vi "case.vi"() -> ()   [LabVIEW 2015]
panel:
  out "Numeric 5":dbl
  in  "Numeric 4":dbl
  out "Numeric 3":dbl
  in  "Boolean":bool
  in  "Numeric 2":dbl
  in  "Numeric":dbl
  # "Case §P§O"
  # "Case §P§O 2"
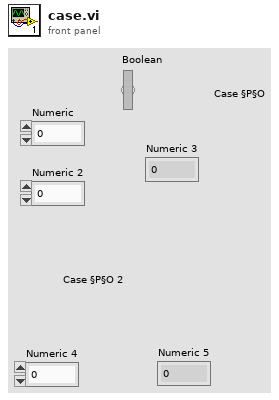
[diagram p1: front panel]
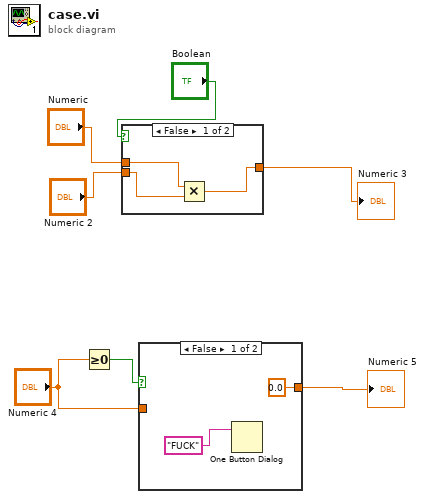
[diagram p0: block diagram]
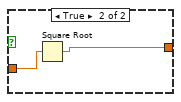
[diagram p2: hidden frame]
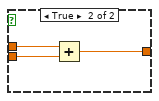
[diagram p3: hidden frame]
diagram:
  n1 = Greater Or Equal To 0?(x="Numeric 4") -> (x >= 0?=w3:bool)
  n2 = case shown="False" "Boolean" {
    tunnel: "Numeric" -> [w10 w13]
    tunnel: "Numeric 2" -> [w9 w12]
    tunnel: [w8 w11] -> w5
    frame False {
      n3 = Multiply(x=w10, y=w9) -> (x*y=w8:dbl)
    }
    frame True {
      n4 = Add(x=w13, y=w12) -> (x+y=w11:dbl)
    }
  }
  "Numeric 3" <- w5
  n5 = case shown="False" w3 {
    tunnel: "Numeric 4" -> [_ w17]
    tunnel: [0.0 w16] -> w1
    frame False {
      n6 = One Button Dialog(message="FUCK") -> ()  [unwired: 1 in, 1 out]
    }
    frame True {
      n7 = Square Root(x=w17) -> (sqrt(x)=w16:dbl)
    }
  }
  "Numeric 5" <- w1
